vi "Send Parameter Message.vi"(5 "Write?":bool, 7 "Param Address":i16, 8 "error in (no error)":errorcluster, 9 "Data":i16, 10 "CAN Offset":u32=160 format="%x", 11 "interface object in":refnum<k20>) -> (0 "error out":errorcluster, 3 "interface object out":refnum<k20>)   [LabVIEW 2014]
uses:
  <vilib>/RioEmbeddedCAN/RioEmbeddedCAN.llb/CANFrameControl.ctl
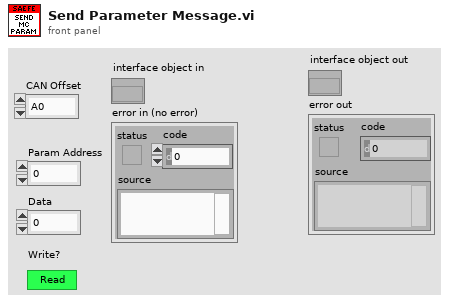
[diagram p1: front panel]
types:
  T1 = typedef "CANFrameControl.ctl" = cluster{"identifier":u32, "extended?":bool, "type":u8, "payload":u8[]}
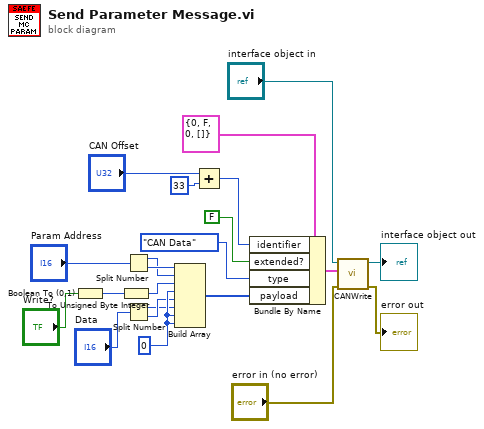
[diagram p0: block diagram]
diagram:
  w14 = u8 0 ("element")
  n1 = Boolean To (0,1)(Boolean="Write?") -> (0, 1=w15:i16)
  n2 = To Unsigned Byte Integer(number=w15) -> (unsigned 8bit integer=w16:u8)
  n3 = Split Number(x="Param Address") -> (hi(x)=w1:u8, lo(x)=w2:u8)
  n4 = Split Number(x="Data") -> (hi(x)=w11:u8, lo(x)=w12:u8)
  n5 = Build Array(w2, w1, w16, w14, w12, w11, w14, w14) -> (w9:u8[])
  n6 = Add(x="CAN Offset", y=u32 33) -> (x+y=w4:u32)
  n7 = Bundle By Name(cluster=T1 {"identifier"=0, "extended?"=FALSE, "type"=0, "payload"=[]} ("CAN frame"), "identifier"=w4, "extended?"=FALSE, "type"=enum8{"CAN Data", "CAN Remote"}."CAN Data", "payload"=w9) -> (w3:T1)
  n8 = call <vilib>:"CANWrite.vi"("error in (no error)"="error in (no error)", "CAN frame"=w3, "interface object in"="interface object in") -> ("error out"=→"error out":errorcluster, "interface object out"=→"interface object out":refnum<k20>)  [unwired: 7 in]
